vi "sub_main_joystick_remote.vi"(8 "error in":errorcluster) -> (0 "error out":errorcluster)   [LabVIEW 2019]
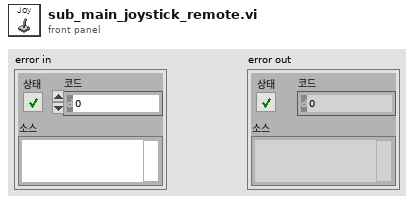
[diagram p1: front panel]
types:
  T1 = cluster{"axis info":cluster{"X axis":i32, "Y axis":i32, "Z axis":i32, "X axis rotation":i32, "Y axis rotation":i32, "Z axis rotation":i32, "U axis":i32, "V axis":i32}, "button info":cluster{"button 1":bool, "button 2":bool, "button 3":bool, "button 4":bool, "button 5":bool, "button 6":bool, "button 7":bool, "button 8":bool, "button 9":bool, "button 10":bool, "button 11":bool, "button 12":bool, "button 13":bool, "button 14":bool, "button 15":bool, "button 16":bool, "button 17":bool, "button 18":bool, "button 19":bool, "button 20":bool, "button 21":bool, "button 22":bool, "button 23":bool, "button 24":bool, "button 25":bool, "button 26":bool, "button 27":bool, "button 28":bool, "button 29":bool, "button 30":bool, "button 31":bool, "button 32":bool}, "direction info":cluster{"pov 1":i32, "pov 2":i32, "pov 3":i32, "pov 4":i32}}
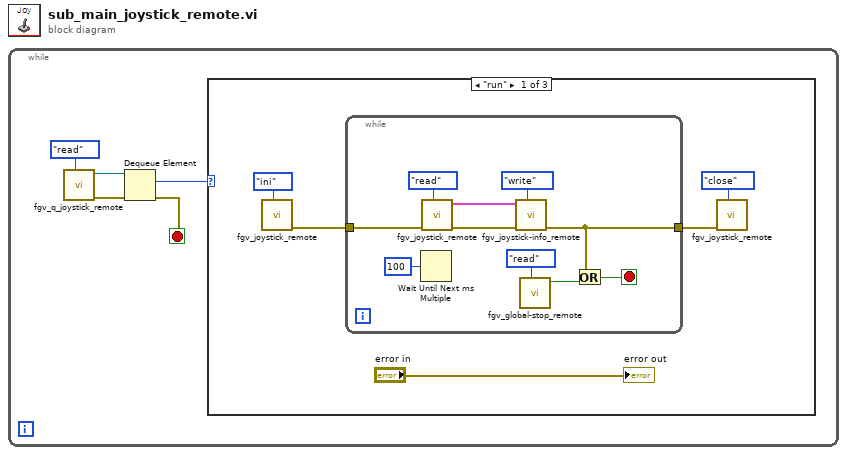
[diagram p0: block diagram]
diagram:
  n1 = while {
    stop <- w4 stop-if-true
    n2 = call "fgv_q_joystick_remote.vi"("cmd"=enum16{"create", "write", "read", "close"}."read") -> ("error out"=w3:errorcluster, "queue out"=w2:refnum<queue>)  [unwired: 9 in]
    n3 = Dequeue Element(queue=w2, error in (no error)=w3) -> (element=w5:enum16{"run", "check", "stop"}, error out=w4:errorcluster)  [unwired: 1 in, 2 out]
    n4 = case shown="\"run\"" w5 {
      frame "run" {
        n5 = call "fgv_joystick_remote.vi"("cmd"=enum16{"ini", "read", "close"}."ini") -> ("error out"=w7:errorcluster)  [unwired: 9 in, 1 out]
        n6 = while {
          tunnel: w7 -> [w14]
          tunnel: [w11] -> w9
          stop <- w20 stop-if-true
          n7 = Wait Until Next ms Multiple(millisecond multiple=u32 100 ("milliseconds to wait")) -> ()  [unwired: 1 out]
          n8 = call "fgv_joystick_remote.vi"("cmd"=enum16{"ini", "read", "close"}."read", "error in"=w14) -> ("error out"=w13:errorcluster, "joystick info-out"=w12:T1)  [unwired: 8 in]
          n9 = call "fgv_joystick-info_remote.vi"("init"=enum16{"enable", "init", "read", "write"}."write", "error in"=w13, "joystick info-in"=w12) -> ("error out"=w11:errorcluster)  [unwired: 5 in, 3 out]
          n10 = call "fgv_global-stop_remote.vi"("cmd"=enum16{"ini", "read", "stop"}."read") -> ("stop status"=w17:bool)  [unwired: 10 in]
          n11 = Or(x=w11, y=w17) -> (x .or. y?=w20:bool)
        }
        n12 = call "fgv_joystick_remote.vi"("cmd"=enum16{"ini", "read", "close"}."close", "error in"=w9) -> ()  [unwired: 8 in, 2 out]
        "error out" <- "error in"
      }
      frame "check" {
      }
      frame "stop", Default {
      }
    }
  }
